vi "Configure Sequencer List Filling.vi"(4 "Level Keep (Off)":bool, 5 "Digital Gain Keep (Off)":bool, 6 "Frequency Keep (Off)":bool, 7 "Range (5)":i32=5, 8 "error in (no error)":errorcluster, 9 "Start Index (1)":i32=1, 10 "Instance (1)":i32=1, 11 "VISA resource name":refnum<visa-resource-name>) -> (0 "error out":errorcluster, 3 "VISA resource name out":refnum<visa-resource-name>)   [LabVIEW 2020, in "Rohde&Schwarz CMXP GPRF.lvlib"]
doc: "Configures settings for filling the list.\n\nAttributes:\nRSCMXPGPRF_ATTR_SEQUENCER_LIST_FILLING_START_INDEX\nRSCMXPGPRF_ATTR_SEQUENCER_LIST_FILLING_RANGE\nRSCMXPGPRF_ATTR_SEQUENCER_LIST_FILLING_FREQUENCY_KEEP\nRSCMXPGPRF_ATTR_SEQUENCER_LIST_FILLING_DIGITAL_GAIN_KEEP\nRSCMXPGPRF_ATTR_SEQUENCER_LIST_FILLING_LEVEL_KEEP\n\nRemote-control commands:\nSOURce:GPRF:GEN<i>:SEQuencer:LIST:FILL:SINDex\nSOURce:GPRF:GEN<i>:SEQuencer:LIST:FILL:RANGe\nSOURce:GPRF:GEN<i>:SEQuencer:LIST:FILL:FREQuency:KEEP\nSOURce:GPRF:GEN<i>:SEQuencer:LIST:FILL:DGAin:KEEP\nSOURce:GPRF:GEN<i>:SEQuencer:LIST:FILL:LRMS:KEEP"
uses:
  <instrlib>/Rohde&Schwarz CMXP GPRF/Rohde&Schwarz CMXP GPRF.lvlib
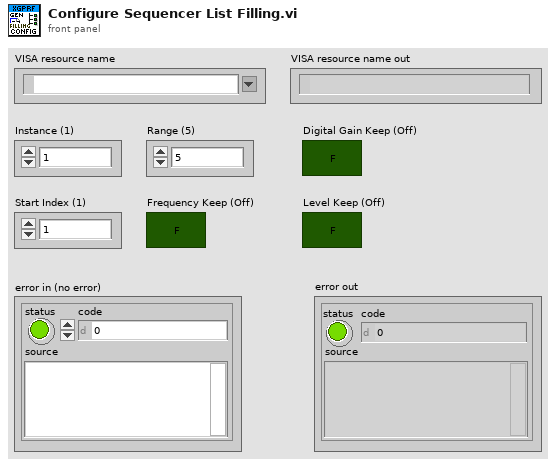
[diagram p1: front panel]
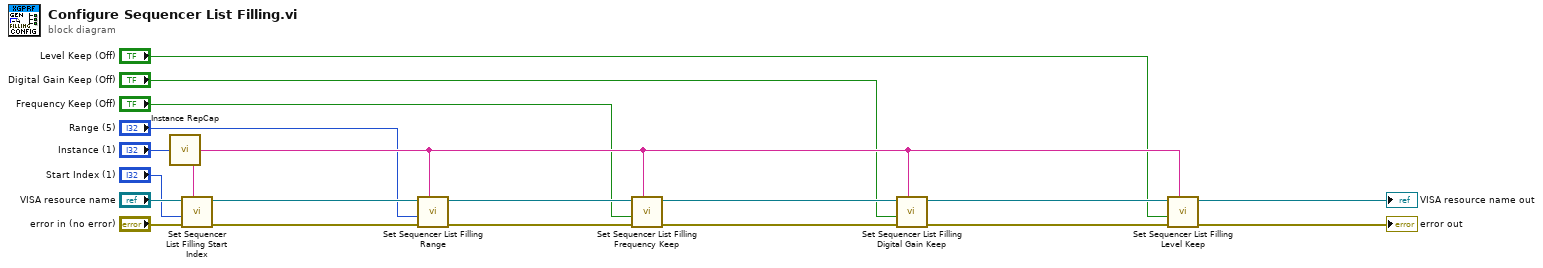
[diagram p0: block diagram]
diagram:
  n1 = call <instrlib>:"Instance RepCap.vi"("Instance in"="Instance (1)") -> ("Instance out"=w6:string)
  n2 = call "Set Sequencer List Filling Start Index"("Repeated Capabilities"=w6, "error in (no error)"="error in (no error)", "Sequencer List Filling Start Index (0)"="Start Index (1)", "instrument handle"="VISA resource name") -> ("error out"=w16:errorcluster, "instrument handle out"=w17:refnum<visa-resource-name>)  [unwired: 6 in]
  n3 = call "Set Sequencer List Filling Range"("Repeated Capabilities"=w6, "error in (no error)"=w16, "Sequencer List Filling Range (0)"="Range (5)", "instrument handle"=w17) -> ("error out"=w14:errorcluster, "instrument handle out"=w15:refnum<visa-resource-name>)  [unwired: 6 in]
  n4 = call "Set Sequencer List Filling Frequency Keep"("Repeated Capabilities"=w6, "error in (no error)"=w14, "Sequencer List Filling Frequency Keep (OFF)"="Frequency Keep (Off)", "instrument handle"=w15) -> ("error out"=w12:errorcluster, "instrument handle out"=w13:refnum<visa-resource-name>)  [unwired: 6 in]
  n5 = call "Set Sequencer List Filling Digital Gain Keep"("Repeated Capabilities"=w6, "error in (no error)"=w12, "Sequencer List Filling Digital Gain Keep (OFF)"="Digital Gain Keep (Off)", "instrument handle"=w13) -> ("error out"=w8:errorcluster, "instrument handle out"=w9:refnum<visa-resource-name>)  [unwired: 6 in]
  n6 = call "Set Sequencer List Filling Level Keep"("Repeated Capabilities"=w6, "error in (no error)"=w8, "Sequencer List Filling Level Keep (OFF)"="Level Keep (Off)", "instrument handle"=w9) -> ("error out"=→"error out":errorcluster, "instrument handle out"=→"VISA resource name out":refnum<visa-resource-name>)  [unwired: 6 in]
